vi "thcd401_query.vi"(6 "delay_sec":dbl caption="Delay Time (s)", 7 "command":string="\n", 8 "error in":errorcluster, 11 "conn_id_in":refnum<k5>) -> (0 "error out":errorcluster, 3 "conn_id_out":refnum<k5>, 4 "status":bool, 5 "data_array":string[](array[string]))   [LabVIEW 2019]
panel:
  out "bytes written":i32
  out "status_read":bool
  out "status_write":bool
  out "command_echo":string
  out "response":string
  out "raw_string":string
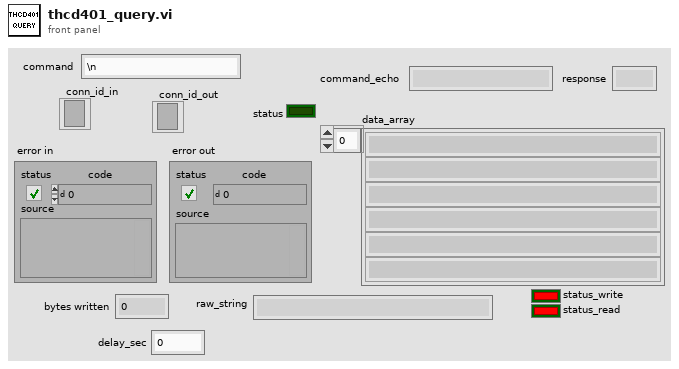
[diagram p1: front panel]
types:
  T1 = enum16{"Standard", "Buffered", "CRLF", "Immediate"}
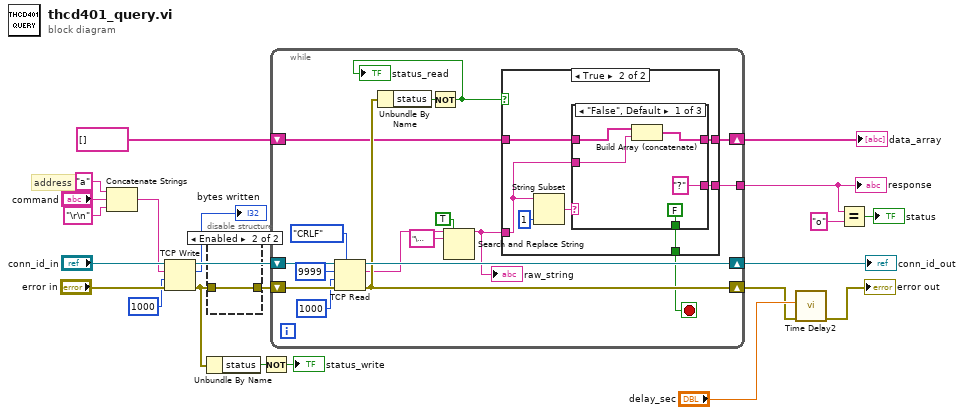
[diagram p0: block diagram]
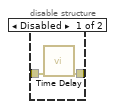
[diagram p2: hidden frame]
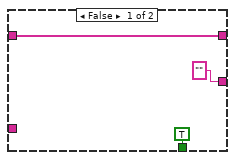
[diagram p3: hidden frame]
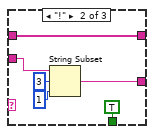
[diagram p4: hidden frame]
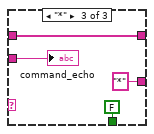
[diagram p5: hidden frame]
diagram:
  # "address"
  n1 = Concatenate Strings("a", "command", "\r\n" ("string")) -> (w17:string)
  n2 = TCP Write(connection ID="conn_id_in", data in=w17, error in (no error)="error in", 9:1000 ("timeout ms (25000)")) -> (connection ID out=w20:refnum<k5>, bytes written=→"bytes written":i32, error out=w7:errorcluster)
  n3 = Unbundle By Name(w7) -> ("status"=w6:bool)
  n4 = disable-structure shown="Enabled" {
    disable-tunnel: w7 -> [w24 w25]
    disable-tunnel: [w23 w25] -> w21
    frame Disabled {
      n5 = call "Time Delay"("error in (no error)"=w24) -> ("error out"=w23:errorcluster)  [unwired: 10 in]
    }
    frame Enabled {
    }
  }
  n6 = Not(x=w6) -> (.not. x?=→"status_write":bool)
  n7 = while {
    shift-right: [w37] -> w2
    shift-left: w21 -> [w42]
    shift-right: [w38] -> w19
    shift-left: w20 -> [w41]
    tunnel: [w36] -> w12
    shift-right: [w34] -> w13
    shift-left: string[] [] ("data_array") -> [w33]
    stop <- w35 stop-if-true
    n8 = TCP Read(connection ID=w41, bytes to read=9999, error in (no error)=w42, 7:T1."CRLF" ("mode (standard)"), 9:1000 ("timeout ms (25000)")) -> (connection ID out=w38:refnum<k5>, data out=w31:string, error out=w37:errorcluster)
    n9 = Unbundle By Name(w37) -> ("status"=w27:bool)
    n10 = Not(x=w27) -> (.not. x?=w26:bool)
    "status_read" <- w26
    n11 = Search and Replace String(replace all?=TRUE ("replace all? (F)"), input string=w31, search string="\u0000") -> (result string=w28:string)  [unwired: 5 in, 3 out]
    "raw_string" <- w28
    n12 = case shown="True" w26 {
      tunnel: w28 -> [_ w50]
      tunnel: ["" ("data out") w49] -> w36
      tunnel: [TRUE w48] -> w35
      tunnel: [w45 w47] -> w34
      tunnel: w33 -> [w45 w46]
      frame False {
      }
      frame True {
        n13 = String Subset(string=w50, length (rest)=1 ("length (rest)")) -> (substring=w51:string)  [unwired: 1 in]
        n14 = case shown="\"False\", Default" w51 {
          tunnel: w50 -> [w54 w63 w64]
          tunnel: ["?" ("data out") w60 "*" ("result string")] -> w49
          tunnel: [FALSE TRUE FALSE] -> w48
          tunnel: [w53 w58 w66] -> w47
          tunnel: w46 -> [w55 w58 w66]
          frame "False", Default {
            n15 = Build Array (concatenate)(w55, w54) -> (w53:string[])
          }
          frame "!" {
            n16 = String Subset(string=w63, offset (0)=3, length (rest)=1 ("length (rest)")) -> (substring=w60:string)
          }
          frame "*" {
            "command_echo" <- w64
          }
        }
      }
    }
  }
  "conn_id_out" <- w19
  "response" <- w12
  "data_array" <- w13
  n17 = call "Time Delay2"("error in (no error)"=w2, "Delay Time (s)"="delay_sec") -> ("error out"=→"error out":errorcluster)  [unwired: 9 in]
  n18 = Equal?(x=w12, y="o") -> (x = y?=→"status":bool)
